vi "Sr830 StatusMessage.vi"() -> (2 "Status Byte Out":bool[](array[boolean]), 3 "message":string=" INSTRUCTIONS:\r\rNormal Use:  When using subVIs that incorporate the error in/error out (or error I/O) structure, place this handler where you want to inform the user of an error, typically at the end of the I/O data path, as the last action of the program.  If the error in error? is ERROR, the handler creates a message describing the error and its source.  If the type of dialog = 1 (default), the message is displayed to the user, who can only acknowedge it.  If the type = 2, the user can acknowledge the message or abort execution; aborting a program with active I/O is not recommended.  If the type = 0, no message is displayed; this is used to process the error programmatically, and the error out cluster elements are wired to individual terminals for that reason.  \r\rOther Use:\n\r\nlocal testing.  To test the error code of a subVI or function that does not have the error I/O structure, you can wire its error code and a source string to the local error code and error source inputs.  If error in error? indicates no error and error code is not equal to 0, the local code and source are substituted for the error in values, and error? is set TRUE (ERROR).")   [LabVIEW 2010]
panel:
  in  "Status Byte":bool[](array[boolean])
  in  "stop":bool
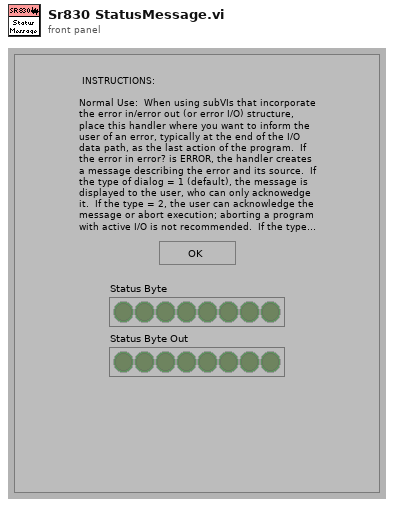
[diagram p1: front panel]
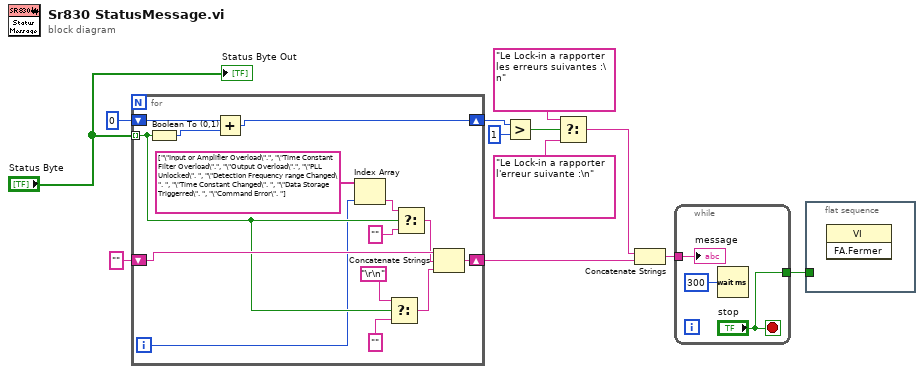
[diagram p0: block diagram]
diagram:
  n1 = for {
    tunnel: "Status Byte" -> [w18] mode=indexing
    shift-right: [w24] -> w11
    shift-left: i16 0 -> [w26]
    shift-right: [w23] -> w4
    shift-left: "" -> [w22]
    i -> [w13]
    n2 = Boolean To (0,1)(Boolean=w18) -> (0, 1=w25:i16)
    n3 = Add(x=w26, y=w25) -> (x+y=w24:i16)
    n4 = Index Array(array=string[] ["\"Input or Amplifier Overload\".", "\"Time Constant Filter Overload\".", "\"Output Overload\".", "\"PLL Unlocked\". ", "\"Detection Frequency range Changed\". ", "\"Time Constant Changed\". ", "\"Data Storage Triggerred\". ", "\"Command Error\". "] ("tableau ajouté"), index=w13) -> (element=w14:string)
    n5 = Select(t="\r\n", s=w18, f="") -> (s? t:f=w15:string)
    n6 = Select(t=w14, s=w18, f="") -> (s? t:f=w20:string)
    n7 = Concatenate Strings(w22, w20, w15) -> (w23:string)
  }
  n8 = Greater?(x=w11, y=i16 1) -> (0:w9:bool)
  n9 = Select(t="Le Lock-in a rapporter les erreurs suivantes :\n" ("message"), s=w9, f="Le Lock-in a rapporter l'erreur suivante :\n" ("message")) -> (s? t:f=w5:string)
  n10 = Concatenate Strings(w5, w4) -> (w3:string)
  n11 = while {
    tunnel: ["stop"] -> w2
    tunnel: w3 -> [w27]
    stop <- "stop" stop-if-true
    n12 = Wait (ms)(milliseconds to wait=u32 300) -> ()  [unwired: 1 out]
    "message" <- w27
  }
  n13 = flat-sequence {
    tunnel: w2 -> [_]
    frame #0 {
      n14 = invoke class="VI" method="FA.Fermer"() -> ()  [unwired: 3 in, 3 out]
    }
  }
  "Status Byte Out" <- "Status Byte"
